vi "main.vi"() -> ()   [LabVIEW 2017]
uses:
  mainVIs/Semaphore.ctl
  mainVIs/States.ctl
panel:
  in  "Pause":bool
  in  "Stop":bool
  out "Semaphore":T1
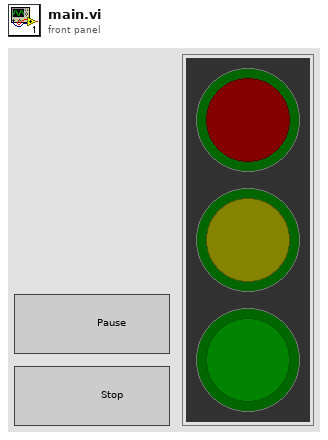
[diagram p1: front panel]
types:
  T1 = typedef "Semaphore.ctl" = cluster{"Red":bool, "Orange":bool, "Green":bool}
  T2 = typedef "States.ctl" = enum16{"Red", "RedAndOrange", "Green", "Orange"}
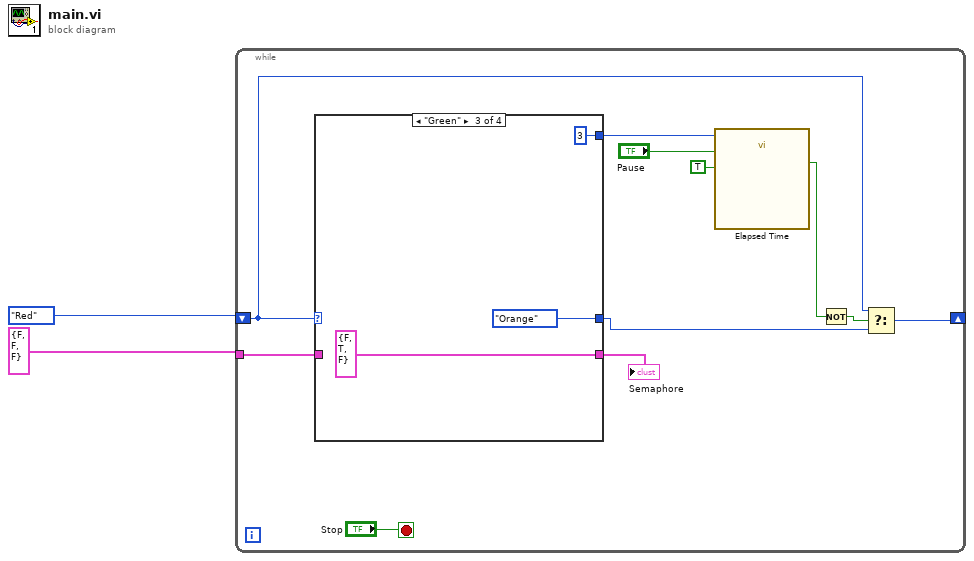
[diagram p0: block diagram]
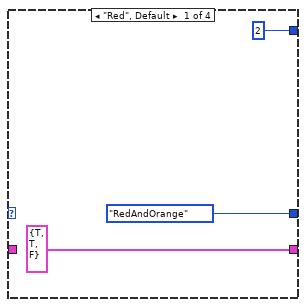
[diagram p2: hidden frame]
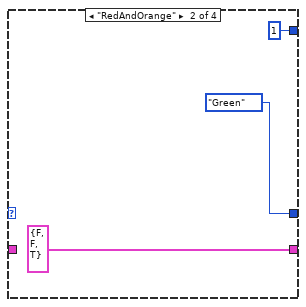
[diagram p3: hidden frame]
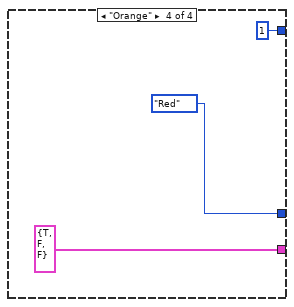
[diagram p4: hidden frame]
diagram:
  n1 = while {
    shift-right: [w9] -> _
    shift-left: States."Red" -> [w8]
    tunnel: T1 {"Red"=FALSE, "Orange"=FALSE, "Green"=FALSE} ("Semaphore") -> [w12]
    stop <- "Stop" stop-if-true
    n2 = case shown="\"Green\"" w8 {
      tunnel: [States."RedAndOrange" States."Green" States."Orange" States."Red"] -> w10
      tunnel: [T1 {"Red"=TRUE, "Orange"=TRUE, "Green"=FALSE} ("Semaphore") T1 {"Red"=FALSE, "Orange"=FALSE, "Green"=TRUE} ("Semaphore") T1 {"Red"=FALSE, "Orange"=TRUE, "Green"=FALSE} ("Semaphore") T1 {"Red"=TRUE, "Orange"=FALSE, "Green"=FALSE} ("Semaphore")] -> w11
      tunnel: w12 -> [_ _ _ _]
      tunnel: [2 1 3 1] -> w7
      frame "Red", Default {
      }
      frame "RedAndOrange" {
      }
      frame "Green" {
      }
      frame "Orange" {
      }
    }
    "Semaphore" <- w11
    n3 = call "Elapsed Time"("Time Target (s)"=w7, "Reset"="Pause", "Auto Reset"=TRUE) -> ("Time has Elapsed"=w3:bool)  [unwired: 9 in, 7 out]
    n4 = Not(x=w3) -> (.not. x?=w4:bool)
    n5 = Select(t=w8, s=w4, f=w10) -> (s? t:f=w9:T2)
  }
